vi "Set discriminator level.vi"(8 "error in (no error)":errorcluster, 9 "Level (-0.034 V)":dbl=-0.034, 10 "Discriminator (def: A)":T1, 11 "VISA resource name":refnum<visa-resource-name>) -> (0 "error out":errorcluster, 3 "VISA resource name out":refnum<visa-resource-name>)   [LabVIEW 2023, in "SR400.lvlib"]
doc: "DL i { ,v }\nThe DL command sets and reads the discriminator\nlevels. i = 0,1, or 2 designates discriminator A,B,\nor T and is required. If v is included, the selected\ndiscriminator level is set to v Volts where -0.3000\n<= V <= 0.3000. The resolution is 0.0002 V (0.2\nmV). If v is absent, the selected discriminator level\nis returned. If the discriminator mode is SCAN,\nthe DL command sets and reads the starting value\nof the level. Changing the level during a scan will\ncause the level to be set to the new value on the\nnext count period. Note that the scan is not reset.\nReading the level during a scan always returns the\nstarting value, not the current value."
uses:
  SR400.lvlib
  Typedefs.llb/Counter.ctl
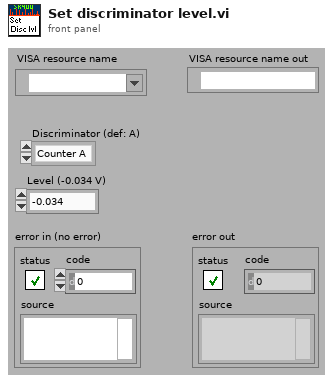
[diagram p1: front panel]
types:
  T1 = typedef "SR400.lvlib/Counter.ctl" = enum16{"Counter A", "Counter B", "Counter T"}
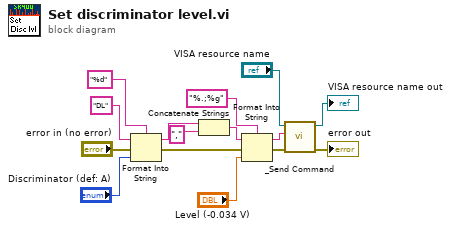
[diagram p0: block diagram]
diagram:
  n1 = Format Into String(format string="%d", initial string="DL" ("command"), error in="error in (no error)", "Discriminator (def: A)") -> (resulting string=w13:string, error out=w14:errorcluster)
  n2 = Concatenate Strings(w13, "," ("command")) -> (w8:string)
  n3 = Format Into String(format string="%.;%g", initial string=w8, error in=w14, "Level (-0.034 V)") -> (resulting string=w5:string, error out=w4:errorcluster)
  n4 = call "_Send Command.vi"("error in (no error)"=w4, "Command"=w5, "VISA resource name"="VISA resource name") -> ("error out"=→"error out":errorcluster, "VISA resource name out"=→"VISA resource name out":refnum<visa-resource-name>)  [unwired: 1 in, 6 out]
